vi "main.vi"() -> ()   [LabVIEW 2025, in "Simple MCP Server.lvlib"]
doc: "This is a simple MCP server demo. Server is started, a tool is added and then the applications stays active and listens for an MCP client to connect and execute the \"Get System Stats.vi\".\n\nTo use the MCP Server, add this code to your claude_desktop_config.json (or other mcp config file for other clients):\n{\n \"mcpServers\": {\n \"vi-scripting-server\": {\n \"command\": \"npx\",\n \"args\": [\n \"mcp-remote\",\n \"http://127.0.0.1:36987/mcp/server\"\n ],\n \"env\": {\n }\n }\n }\n}"
uses:
  Simple MCP Server.lvlib
  src/MCP Server/MCP Server.lvlib
panel:
  in  "stop":bool
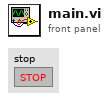
[diagram p1: front panel]
types:
  T1 = typedef "MCP Server.lvlib/User Events.ctl" = cluster{"onError":refnum<user-event>, "onRpc":refnum<user-event>}
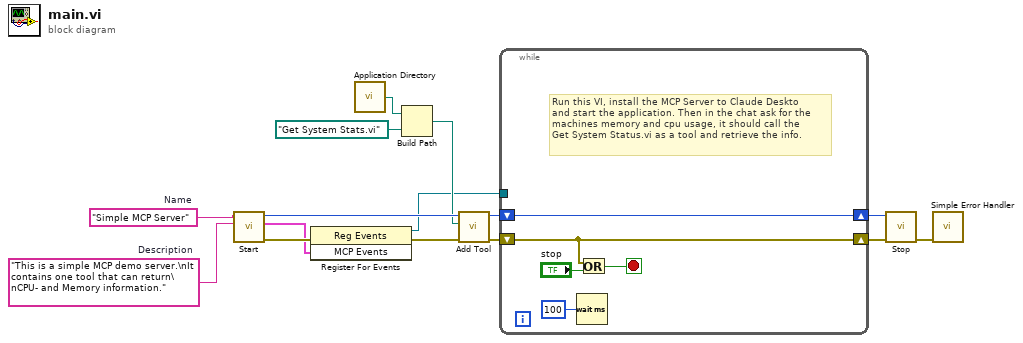
[diagram p0: block diagram]
diagram:
  w8 = "This is a simple MCP demo server.\nIt contains one tool that can return\nCPU- and Memory information."  # Description
  w9 = "Simple MCP Server"  # Name
  n1 = call "Start.vi"("Description"=w8, "Name"=w9) -> ("error out"=w15:errorcluster, "MCP Events"=w1:T1, "server id out"=w14:i32)  [unwired: 7 in]
  n2 = register-events(error in=w15, w1) -> (reference out=w2:refnum<event-registration>, error out=w3:errorcluster)  [unwired: 1 in]
  n3 = call <vilib>:"Application Directory.vi"() -> ("Application Directory"=w7:path)
  n4 = Build Path(base path=w7, name or relative path=path "Get System Stats.vi") -> (appended path=w5:path)
  n5 = call "Add Tool.vi"("error in (no error)"=w3, "vi path"=w5, "server id"=w14) -> ("error out"=w13:errorcluster, "server id out"=w11:i32)  [unwired: 7 in]
  n6 = while {
    shift-right: [w17] -> w12
    shift-left: w13 -> [w17]
    shift-right: [w20] -> w10
    shift-left: w11 -> [w20]
    tunnel: w2 -> [_]
    stop <- w18 stop-if-true
    # "Run this VI, install the MCP Server to Claude Deskto\nand start the application. Then in the chat ask for the\nmachines memory and cpu usage, it should call the \nGet System Status.vi as a tool and retrieve the info."
    n7 = Wait (ms)(milliseconds to wait=u32 100) -> ()  [unwired: 1 out]
    n8 = Or(x=w17, y="stop") -> (x .or. y?=w18:bool)
  }
  n9 = call "Stop.vi"("error in (no error)"=w12, "id"=w10) -> ("error out"=w4:errorcluster)  [unwired: 9 in]
  n10 = call <vilib>:"Simple Error Handler.vi"("error in (no error)"=w4) -> ()  [unwired: 4 in, 5 out]
